vi "Cluster.vi"() -> ()   [LabVIEW 2022 SP3]
panel:
  out "String 6":string
  out "String 5":string
  out "error out":errorcluster
  in  "file (use dialog)":path
  out "output cluster 3":cluster{"Numeric":dbl, "String":string}
  out "output cluster 2":cluster{"String":string}
  out "output cluster":T1
  in  "String 4":string
  in  "Numeric 5":dbl
  in  "Numeric 4":dbl
  out "String 3":string
  out "Numeric 3":dbl
  out "String 2":string
  out "String":string
  out "Boolean":bool
  out "Numeric 2":dbl
  out "Numeric":dbl
  in  "Cluster 3":cluster{"Numeric":dbl, "String":string}
  in  "Cluster 2":cluster{"String":string}
  in  "Cluster":T2
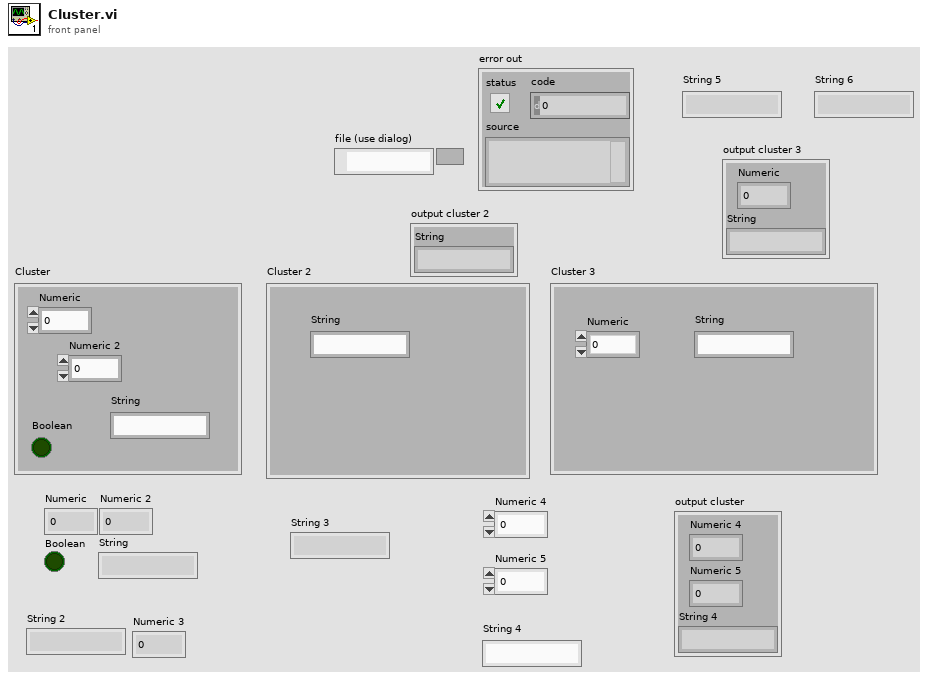
[diagram p1: front panel]
types:
  T1 = cluster{"Numeric 4":dbl, "Numeric 5":dbl, "String 4":string}
  T2 = cluster{"Numeric":dbl, "Numeric 2":dbl, "Boolean":bool, "String":string}
  T3 = cluster{"Integer":i32, "Double":dbl, "String":string}
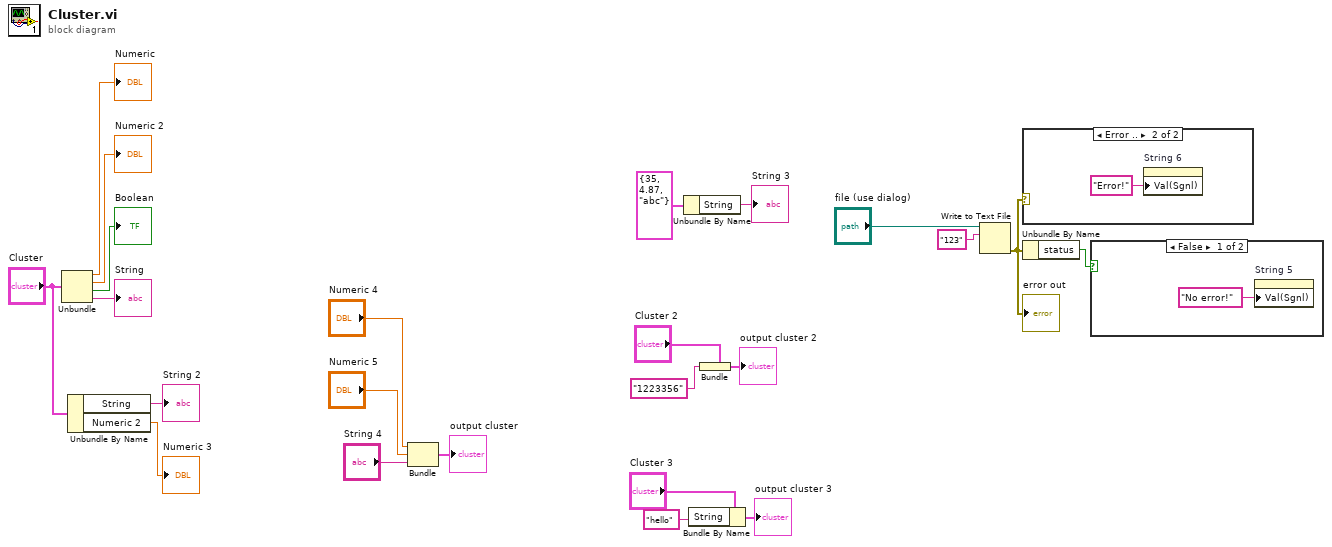
[diagram p0: block diagram]
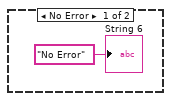
[diagram p2: hidden frame]
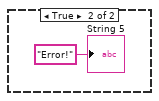
[diagram p3: hidden frame]
diagram:
  n1 = Unbundle("Cluster") -> ("Numeric"=→"Numeric":dbl, "Numeric 2"=→"Numeric 2":dbl, "Boolean"=→"Boolean":bool, "String"=→"String":string)
  n2 = Unbundle By Name("Cluster") -> ("String"=→"String 2":string, "Numeric 2"=→"Numeric 3":dbl)
  n3 = Bundle("Numeric 4"="Numeric 4", "Numeric 5"="Numeric 5", "String 4"="String 4") -> (→"output cluster":T1)  [unwired: 1 in]
  n4 = Unbundle By Name(T3 {"Integer"=35, "Double"=4.87, "String"="abc"}) -> ("String"=→"String 3":string)
  n5 = Bundle By Name(cluster="Cluster 3", "String"="hello") -> (→"output cluster 3":cluster{"Numeric":dbl, "String":string})
  n6 = Bundle(cluster="Cluster 2", "String"="1223356") -> (→"output cluster 2":cluster{"String":string})
  n7 = Write to Text File(file (use dialog)="file (use dialog)", text="123") -> (error out=w1:errorcluster)  [unwired: 2 in, 2 out]
  "error out" <- w1
  n8 = case shown="Error .." w1 {
    frame No Error {
      "String 6" <- "No Error" ("String 6")
    }
    frame Error {
      n9 = property on="String 6" class="Str"("Val(Sgnl)"="Error!" ("Value (Signaling)")) -> ()  [unwired: 2 in, 2 out]
    }
  }
  n10 = Unbundle By Name(w1) -> ("status"=w2:bool)
  n11 = case shown="False" w2 {
    frame False {
      n12 = property on="String 5" class="Str"("Val(Sgnl)"="No error!" ("Value (Signaling)")) -> ()  [unwired: 2 in, 2 out]
    }
    frame True {
      "String 5" <- "Error!" ("String 5")
    }
  }
